vi "LocalQuadraticSum.vi"   [LabVIEW 2014]
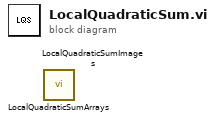
[diagram p0: block diagram]
diagram:
  n1 = call "LocalQuadraticSumArrays.vi"() -> ()  [unwired: 11 in, 1 out]
  n2 = call "LocalQuadraticSumImages.vi"() -> ()  [unwired: 11 in, 1 out]
